vi "To String (Array).vi"(6 "pretty print? (T)":bool=TRUE, 7 "enable LabVIEW extensions? (T)":bool=TRUE, 8 "error in (no error)":errorcluster, 10 "indent":i32, 11 "JSON Value in":refnum<class "JSON Value.lvclass">) -> (0 "error out":errorcluster, 3 "String":string)   [LabVIEW 2016, in "JSON Value.lvclass"]
doc: "Flattens the given JSON data to a string."
uses:
  JSON Value.lvclass
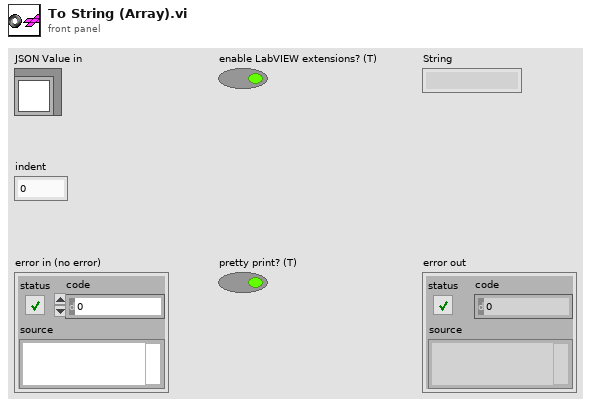
[diagram p1: front panel]
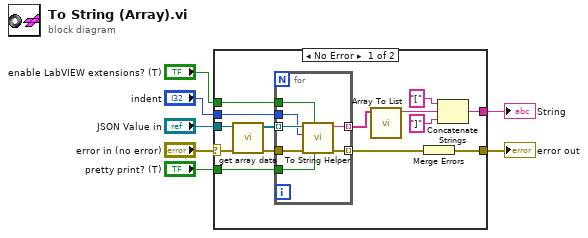
[diagram p0: block diagram]
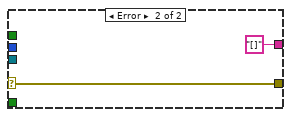
[diagram p2: hidden frame]
diagram:
  n1 = case shown="No Error" "error in (no error)" {
    selector: "error in (no error)" -> [w11 w30]
    tunnel: "JSON Value in" -> [w13 _]
    tunnel: [w19 w30] -> w5
    tunnel: [w18 "[]"] -> w4
    tunnel: "enable LabVIEW extensions? (T)" -> [w14 _]
    tunnel: "pretty print? (T)" -> [w9 _]
    tunnel: "indent" -> [w8 _]
    frame No Error {
      n2 = call "get array data.vi"("error in (no error)"=w11, "JSON Value in"=w13) -> ("error out"=w10:errorcluster, "JSON Array out"=w12:refnum<class "JSON Value.lvclass">[])  [unwired: 8 in]
      n3 = for {
        tunnel: [w28] -> w21 mode=indexing
        tunnel: w10 -> [w27]
        tunnel: [w26] -> w20 mode=indexing
        tunnel: w14 -> [w25]
        tunnel: w12 -> [w24] mode=indexing
        tunnel: w9 -> [w23]
        tunnel: w8 -> [w22]
        n4 = call "To String Helper.vi"("pretty print? (T)"=w23, "enable LabVIEW extensions? (T)"=w25, "error in (no error)"=w27, "indent"=w22, "JSON Value in"=w24) -> ("error out"=w26:errorcluster, "String"=w28:string)  [unwired: 5 in]
      }
      n5 = call "Array To List.vi"("Array"=w21) -> ("String"=w17:string)  [unwired: 10 in]
      n6 = Merge Errors(w20) -> (w19:errorcluster)
      n7 = Concatenate Strings("[" ("string"), w17, "]" ("string")) -> (w18:string)
    }
    frame Error {
    }
  }
  "String" <- w4
  "error out" <- w5
